vi "Modem Status Interface settings.vi"(1 "Action(GET)":enum16{"GET", "SET"}(ring), 7 "Modem Status VISA  name  in":refnum<visa-resource-name>, 11 "error in (no error)":errorcluster) -> (8 "PCP VISA  name  out":refnum<visa-resource-name>, 10 "baud rate out":u32, 15 "error out":errorcluster)   [LabVIEW 2011]
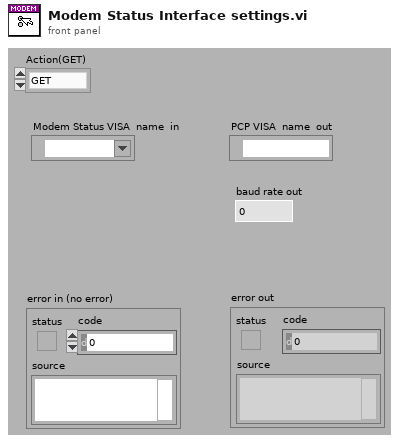
[diagram p1: front panel]
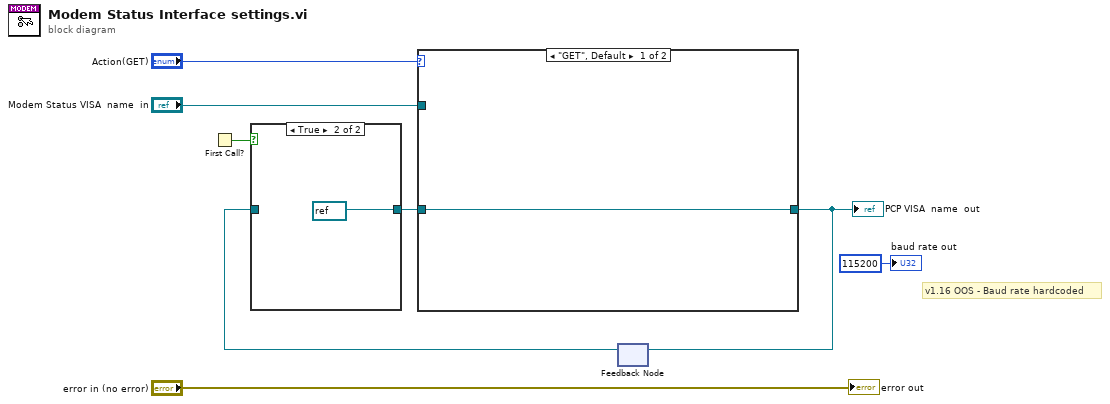
[diagram p0: block diagram]
diagram:
  # "v1.16 OOS - Baud rate hardcoded"
  n1 = First Call?() -> (First Call?: T/F=w5:bool)
  n2 = feedback #1() -> (w6:refnum<visa-resource-name>)  [unwired: 1 in]
  n3 = case shown="True" w5 {
    tunnel: w6 -> [w9 _]
    tunnel: [w9 refnum<visa-resource-name> refnum ("PCP VISA  name")] -> w3
    frame False {
    }
    frame True {
    }
  }
  n4 = case shown="\"GET\", Default" "Action(GET)" {
    tunnel: [w11 w12] -> w4
    tunnel: w3 -> [w11 _]
    tunnel: "Modem Status VISA  name  in" -> [_ w12]
    frame "GET", Default {
    }
    frame "SET" {
    }
  }
  "PCP VISA  name  out" <- w4
  n5 = feedback-in #1(w4) -> ()
  "error out" <- "error in (no error)"
  "baud rate out" <- u32 115200 ("baud rate out")
